vi "getDevAttributesFromTree.vi"(8 "error in (no error)":errorcluster, 9 "Cluster in":T1, 10 "Tree pics & devs in":string, 11 "TreeControl in":refnum<vi>) -> (0 "error out":errorcluster, 3 "Cluster out":T1)   [LabVIEW 2013, in "DataCreation.lvlib"]
uses:
  DataCreation.lvlib
  vis/SetupData2.ctl
  classes/Datastructure/Device/Device.lvclass
  classes/Datastructure/Image/img.lvclass
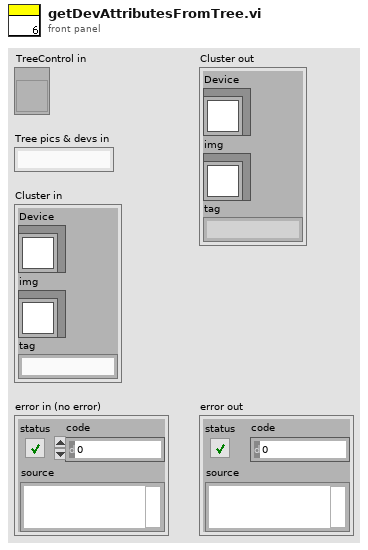
[diagram p1: front panel]
types:
  T1 = typedef "SetupData2.ctl" = cluster{"Device":refnum<class "Device.lvclass">, "img":refnum<class "img.lvclass">, "tag":string}
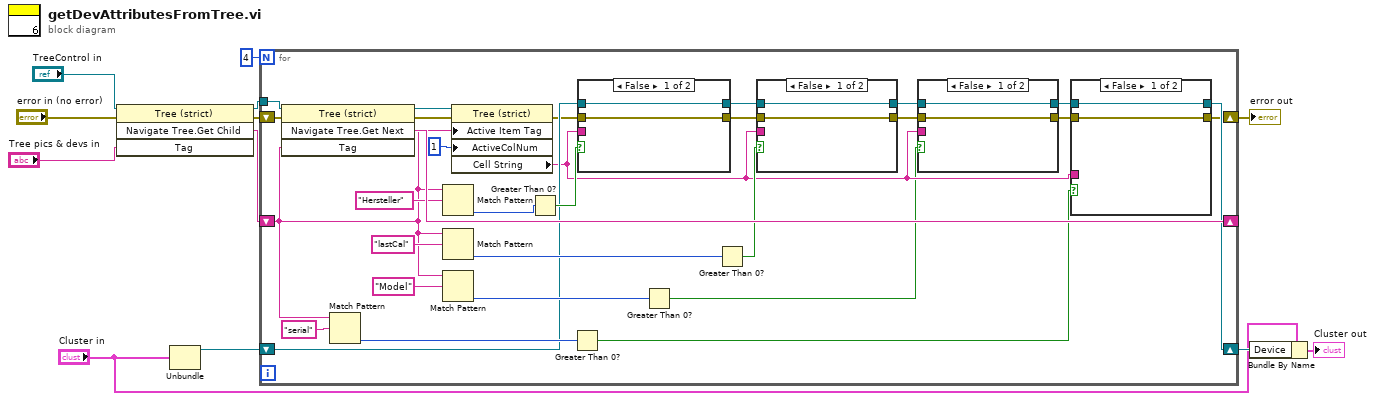
[diagram p0: block diagram]
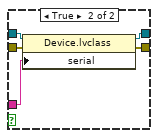
[diagram p2: hidden frame]
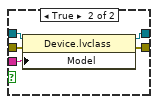
[diagram p3: hidden frame]
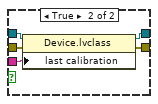
[diagram p4: hidden frame]
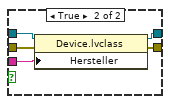
[diagram p5: hidden frame]
diagram:
  n1 = invoke class="Tree (strict)" method="Navigate Tree.Get Child"(reference="TreeControl in", error in="error in (no error)", "Tag"="Tree pics & devs in") -> (reference out=w5:refnum<vi>, error out=w8:errorcluster, "Navigate Tree:Get Child"=w1:string)  [unwired: 1 in, 1 out]
  n2 = Unbundle("Cluster in") -> ("Device"=w9:refnum<class "Device.lvclass">)  [unwired: 2 out]
  n3 = for {
    N: 4 -> [_]
    tunnel: w5 -> [w23]
    shift-right: [w42] -> _
    shift-left: w1 -> [w31]
    shift-right: [w15] -> w11
    shift-left: w8 -> [w24]
    shift-right: [w25] -> w10
    shift-left: w9 -> [w29]
    n4 = invoke class="Tree (strict)" method="Navigate Tree.Get Next"(reference=w23, error in=w24, "Tag"=w31) -> (reference out=w16:refnum<vi>, error out=w20:errorcluster, "Navigate Tree:Get Next Item"=w42:string)  [unwired: 1 in, 1 out]
    n5 = Match Pattern(string=w31, regular expression="serial" ("Linker Zellen-String")) -> (offset past match=w36:i32)  [unwired: 1 in, 3 out]
    n6 = Match Pattern(string=w31, regular expression="Hersteller" ("Left Cell String")) -> (offset past match=w39:i32)  [unwired: 1 in, 3 out]
    n7 = Match Pattern(string=w31, regular expression="lastCal" ("Linker Zellen-String")) -> (offset past match=w37:i32)  [unwired: 1 in, 3 out]
    n8 = Match Pattern(string=w31, regular expression="Model" ("Linker Zellen-String")) -> (offset past match=w35:i32)  [unwired: 1 in, 3 out]
    n9 = property class="Tree (strict)"(reference=w16, error in=w20, "Active Item Tag"=w31, "ActiveColNum"=1 ("Active Cell:Active Column Number")) -> (error out=w17:errorcluster, "Cell String"=w18:string)  [unwired: 1 out]
    n10 = Greater Than 0?(x=w39) -> (x > 0?=w40:bool)
    n11 = Greater Than 0?(x=w36) -> (x > 0?=w14:bool)
    n12 = case shown="False" w40 {
      tunnel: w17 -> [w64 w70]
      tunnel: [w64 w69] -> w19
      tunnel: w29 -> [w65 w68]
      tunnel: [w65 w67] -> w28
      tunnel: w18 -> [_ w66]
      frame False {
      }
      frame True {
        n13 = property class="Device.lvclass"(reference=w68, error in=w70, "Hersteller"=w66) -> (reference out=w67:refnum<class "Device.lvclass">, error out=w69:errorcluster)
      }
    }
    n14 = Greater Than 0?(x=w35) -> (x > 0?=w13:bool)
    n15 = Greater Than 0?(x=w37) -> (x > 0?=w30:bool)
    n16 = case shown="False" w30 {
      tunnel: w19 -> [w57 w63]
      tunnel: [w57 w62] -> w22
      tunnel: w28 -> [w58 w61]
      tunnel: [w58 w60] -> w27
      tunnel: w18 -> [_ w59]
      frame False {
      }
      frame True {
        n17 = property class="Device.lvclass"(reference=w61, error in=w63, "last calibration"=w59) -> (reference out=w60:refnum<class "Device.lvclass">, error out=w62:errorcluster)
      }
    }
    n18 = case shown="False" w13 {
      tunnel: w22 -> [w50 w56]
      tunnel: [w50 w55] -> w21
      tunnel: w27 -> [w51 w54]
      tunnel: [w51 w53] -> w26
      tunnel: w18 -> [_ w52]
      frame False {
      }
      frame True {
        n19 = property class="Device.lvclass"(reference=w54, error in=w56, "Model"=w52) -> (reference out=w53:refnum<class "Device.lvclass">, error out=w55:errorcluster)
      }
    }
    n20 = case shown="False" w14 {
      tunnel: w21 -> [w43 w49]
      tunnel: [w43 w48] -> w15
      tunnel: w26 -> [w44 w47]
      tunnel: [w44 w46] -> w25
      tunnel: w18 -> [_ w45]
      frame False {
      }
      frame True {
        n21 = property class="Device.lvclass"(reference=w47, error in=w49, "serial"=w45) -> (reference out=w46:refnum<class "Device.lvclass">, error out=w48:errorcluster)
      }
    }
  }
  "error out" <- w11
  n22 = Bundle By Name(cluster="Cluster in", "Device"=w10) -> (→"Cluster out":T1)
